vi "launcher.vi"   [LabVIEW 2025]
uses:
  root_actor/root_actor/root_actor.lvclass
  Applications/National Instruments/LabVIEW 2025 64-bit/vi.lib/ActorFramework/Actor/Actor.lvclass
  <vilib>/ActorFramework/Actor/Actor.lvclass
panel:
  # "LAUNCHER"
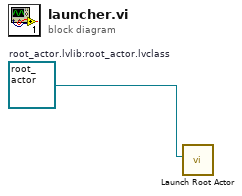
[diagram p0: block diagram]
diagram:
  w1 = refnum<class "root_actor.lvclass"> refnum  # root_actor.lvlib:root_actor.lvclass
  n1 = call <vilib>:"Launch Root Actor.vi"("Actor"=w1) -> ()  [unwired: 9 in, 2 out]
